vi "DG1022General.vi"() -> ()   [LabVIEW 2021]
panel:
  in  "Output 1":bool
  in  "Output 2":bool
  out "output control error":errorcluster
  in  "Stop Button":bool
  in  "VISA resource name":refnum<visa-resource-name>
  in  "Frequency (1000 Hz)":dbl=1000.0
  in  "Unit (0: Vpp)":u16
  in  "DC Offset (0.00 V)":dbl
  in  "Amplitude (1)":dbl=1.0
  in  "Waveform Function (1: Sine)":u16(ring)=1 items=["DC", "Sine", "Square", "Ramp", "Pulse", "Noise", "Sinc", "Negative Ramp", "Exponential Rise", "Exponential Fall", "Cardiac"]
  in  "Configure":bool
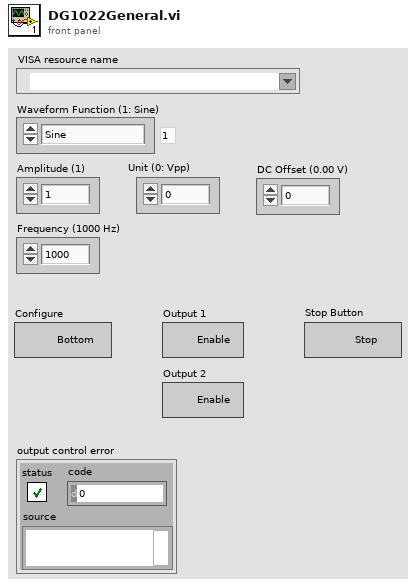
[diagram p1: front panel]
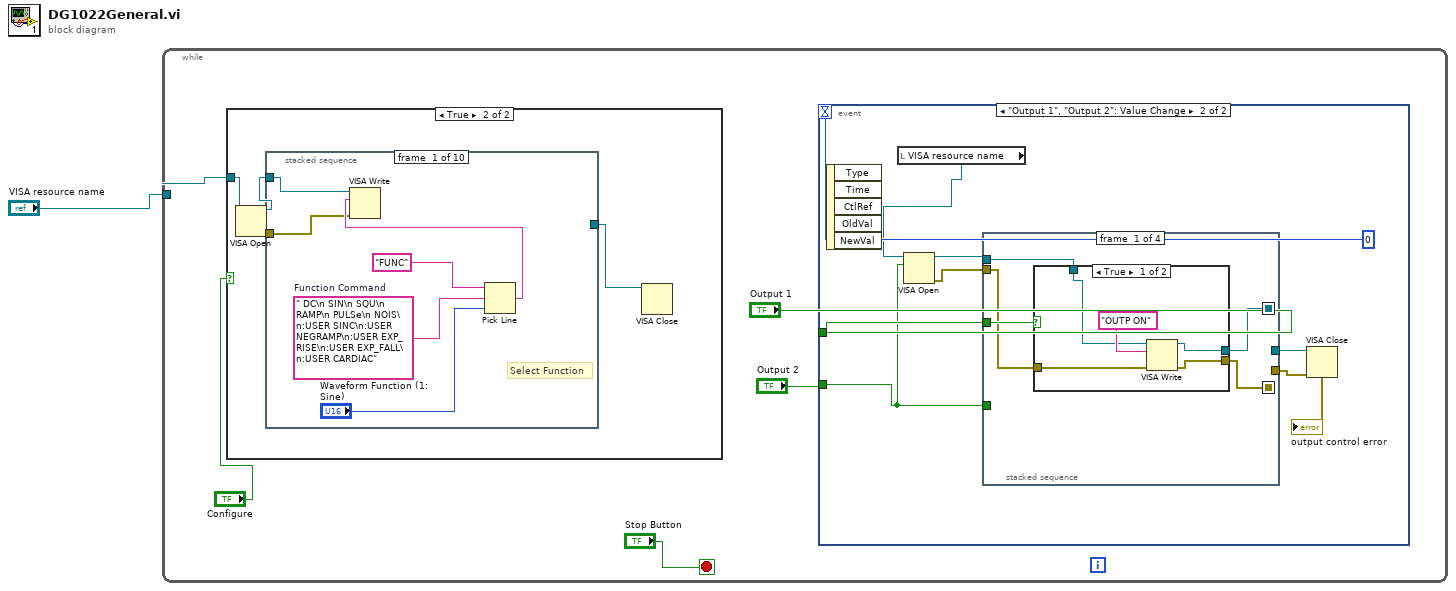
[diagram p0: block diagram]
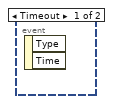
[diagram p2: hidden frame]
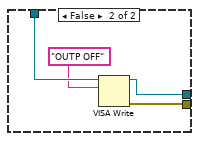
[diagram p3: hidden frame]
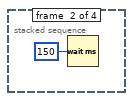
[diagram p4: hidden frame]
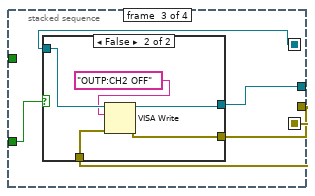
[diagram p5: hidden frame]
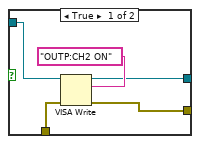
[diagram p6: hidden frame]
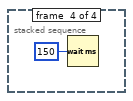
[diagram p7: hidden frame]
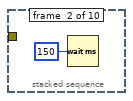
[diagram p9: hidden frame]
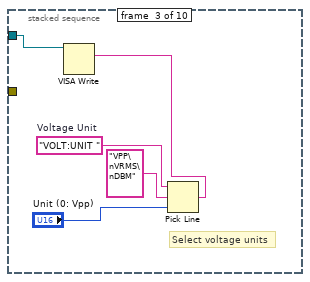
[diagram p10: hidden frame]
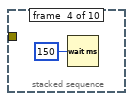
[diagram p11: hidden frame]
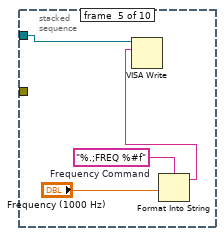
[diagram p12: hidden frame]
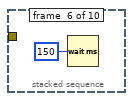
[diagram p13: hidden frame]
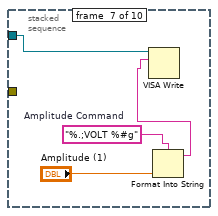
[diagram p14: hidden frame]
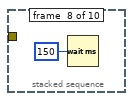
[diagram p15: hidden frame]
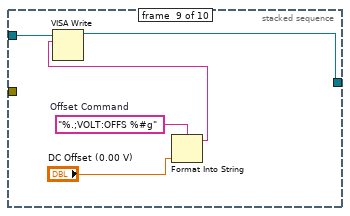
[diagram p16: hidden frame]
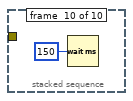
[diagram p17: hidden frame]
diagram:
  n1 = while {
    tunnel: "VISA resource name" -> [w7]
    stop <- "Stop Button" stop-if-true
    n2 = case shown="True" "Configure" {
      tunnel: w7 -> [_ w49]
      frame False {
      }
      frame True {
        n3 = VISA Open(VISA resource name=w49) -> (VISA resource name=w50:refnum<visa-resource-name>, error out=w48:errorcluster)  [unwired: 4 in]
        n4 = stacked-sequence {
          tunnel: w50 -> [w54 _ w59 _ w66 _ w70 _ w77 _]
          tunnel: w48 -> [w51 _ _ _ _ _ _ _ _ _]
          tunnel: [_ _ _ _ _ _ _ _ w74 _] -> w47
          frame #0 {
            w53 = " DC\n SIN\n SQU\n RAMP\n PULSe\n NOIS\n:USER SINC\n:USER NEGRAMP\n:USER EXP_RISE\n:USER EXP_FALL\n:USER CARDIAC"  # Function Command
            # "Select Function"
            n5 = Pick Line(string ("")="FUNC", multi-line string=w53, line index="Waveform Function (1: Sine)") -> (output string=w55:string)
            n6 = VISA Write(VISA resource name=w54, write buffer=w55, error in (no error)=w51) -> ()  [unwired: 3 out]
          }
          frame #1 {
            n7 = Wait (ms)(milliseconds to wait=u32 150) -> ()  [unwired: 1 out]
          }
          frame #2 {
            w61 = "VOLT:UNIT "  # Voltage Unit
            # "Select voltage units"
            n8 = Pick Line(string ("")=w61, multi-line string="VPP\nVRMS\nDBM", line index="Unit (0: Vpp)") -> (output string=w60:string)
            n9 = VISA Write(VISA resource name=w59, write buffer=w60) -> ()  [unwired: 1 in, 3 out]
          }
          frame #3 {
            n10 = Wait (ms)(milliseconds to wait=u32 150) -> ()  [unwired: 1 out]
          }
          frame #4 {
            w67 = "%.;FREQ %#f"  # Frequency Command
            n11 = Format Into String(format string=w67, "Frequency (1000 Hz)") -> (resulting string=w65:string)  [unwired: 2 in, 1 out]
            n12 = VISA Write(VISA resource name=w66, write buffer=w65) -> ()  [unwired: 1 in, 3 out]
          }
          frame #5 {
            n13 = Wait (ms)(milliseconds to wait=u32 150) -> ()  [unwired: 1 out]
          }
          frame #6 {
            w71 = "%.;VOLT %#g"  # Amplitude Command
            n14 = Format Into String(format string=w71, "Amplitude (1)") -> (resulting string=w72:string)  [unwired: 2 in, 1 out]
            n15 = VISA Write(VISA resource name=w70, write buffer=w72) -> ()  [unwired: 1 in, 3 out]
          }
          frame #7 {
            n16 = Wait (ms)(milliseconds to wait=u32 150) -> ()  [unwired: 1 out]
          }
          frame #8 {
            w78 = "%.;VOLT:OFFS %#g"  # Offset Command
            n17 = Format Into String(format string=w78, "DC Offset (0.00 V)") -> (resulting string=w76:string)  [unwired: 2 in, 1 out]
            n18 = VISA Write(VISA resource name=w77, write buffer=w76) -> (VISA resource name out=w74:refnum<visa-resource-name>)  [unwired: 1 in, 2 out]
          }
          frame #9 {
            n19 = Wait (ms)(milliseconds to wait=u32 150) -> ()  [unwired: 1 out]
          }
        }
        n20 = VISA Close(VISA resource name=w47) -> ()  [unwired: 1 in, 1 out]
      }
    }
    n21 = event shown="[1] \"Output 1\", \"Output 2\": Value Change" {
      selector: _ -> [_ _]
      dyn-events: _ -> [_ _]
      timeout: u32 0 ("Time") -> [_ _]
      tunnel: "Output 2" -> [_ w8]
      tunnel: "Output 1" -> [_ w15]
      event Timeout {
        n22 = event-data() -> ()  [unwired: 1 in, 2 out]
      }
      event "Output 1", "Output 2": Value Change {
        n23 = event-data() -> ()  [unwired: 1 in, 5 out]
        n24 = local read "VISA resource name"() -> (w9:refnum<visa-resource-name>)
        n25 = VISA Open(duplicate session (F)=w8, VISA resource name=w9) -> (VISA resource name=w14:refnum<visa-resource-name>, error out=w13:errorcluster)  [unwired: 3 in]
        n26 = stacked-sequence {
          seq-local: [w18 _ _ _] -> [_ _ w34 _]
          seq-local: [w16 _ _ _] -> [_ _ w32 _]
          tunnel: w14 -> [w20 _ _ _]
          tunnel: w8 -> [_ _ w35 _]
          tunnel: w15 -> [w19 _ _ _]
          tunnel: [_ _ w33 _] -> w12
          tunnel: w13 -> [w17 _ _ _]
          tunnel: [_ _ w31 _] -> w11
          frame #0 {
            n27 = case shown="True" w19 {
              tunnel: w20 -> [w24 w29]
              tunnel: [w23 w27] -> w18
              tunnel: w17 -> [w22 _]
              tunnel: [w21 w26] -> w16
              frame True {
                n28 = VISA Write(VISA resource name=w24, write buffer="OUTP ON", error in (no error)=w22) -> (VISA resource name out=w21:refnum<visa-resource-name>, error out=w23:errorcluster)  [unwired: 1 out]
              }
              frame False {
                n29 = VISA Write(VISA resource name=w29, write buffer="OUTP OFF") -> (VISA resource name out=w26:refnum<visa-resource-name>, error out=w27:errorcluster)  [unwired: 1 in, 1 out]
              }
            }
          }
          frame #1 {
            n30 = Wait (ms)(milliseconds to wait=u32 150) -> ()  [unwired: 1 out]
          }
          frame #2 {
            n31 = case shown="False" w35 {
              tunnel: w32 -> [w39 w45]
              tunnel: [w38 w43] -> w33
              tunnel: w34 -> [w37 w42]
              tunnel: [w36 w41] -> w31
              frame True {
                n32 = VISA Write(VISA resource name=w39, write buffer="OUTP:CH2 ON", error in (no error)=w37) -> (VISA resource name out=w36:refnum<visa-resource-name>, error out=w38:errorcluster)  [unwired: 1 out]
              }
              frame False {
                n33 = VISA Write(VISA resource name=w45, write buffer="OUTP:CH2 OFF", error in (no error)=w42) -> (VISA resource name out=w41:refnum<visa-resource-name>, error out=w43:errorcluster)  [unwired: 1 out]
              }
            }
          }
          frame #3 {
            n34 = Wait (ms)(milliseconds to wait=u32 150) -> ()  [unwired: 1 out]
          }
        }
        n35 = VISA Close(VISA resource name=w11, error in (no error)=w12) -> (error out=→"output control error":errorcluster)
      }
    }
  }
